vi "Rd Wr Focus settings json.vi"(7 "Focus Name":string="Default", 8 "error in (no error)":errorcluster, 9 "Settings File":string="CC System Settings.json", 10 "Write? (F:Read)":bool, 11 "Focus Settings":T1) -> (0 "error out":errorcluster, 3 "Focus Settings":T1)   [LabVIEW 2024]
uses:
  Focus cluster Settings.ctl
  Focus Hardware Types.ctl
  Focus cluster Motion Settings.ctl
  2e80df6d-94aa-46b9-8b94-ceea8c057880.vi
  659fb017-0e9f-42f9-b06e-930303f00cbc.vi
  <vilib>/JDP Science/JSONtext/Find Item.vi
  <vilib>/JDP Science/JSONtext/Next JSON Value.vi
  <vilib>/JDP Science/JSONtext/String Subset.vi
  <vilib>/JDP Science/JSONtext/Parsing/Advance past next JSON Value (inlined COPY).vi
  <vilib>/JDP Science/JSONtext/Parsing/Advance past whitespace.vi
  <vilib>/JDP Science/JSONtext/Parsing/Advance past String.vi
  <vilib>/JDP Science/JSONtext/Parsing/Advance past Number.vi
  <vilib>/JDP Science/JSONtext/Parsing/Advance past Line Ending.vi
  <vilib>/JDP Science/JSONtext/Parsing/Parse Full Path or Item Name.vi
  <vilib>/JDP Science/JSONtext/Parsing/Advance past Array.vi
  <vilib>/JDP Science/JSONtext/Parsing/Advance past Object.vi
  <vilib>/JDP Science/JSONtext/support/Error Cluster From Code.vi
  <vilib>/JDP Science/JSONtext/Offset/Find Item Locations by Path.vi
  <vilib>/JDP Science/JSONtext/JSON text to Variant.vi
  <vilib>/JDP Science/JSONtext/Variant to JSON Text.vi
  <vilib>/JDP Science/JSONtext/Set Item.vi
  <vilib>/JDP Science/JSONtext/LVClass Serializer/JSONtext LVClass Serializer.lvclass
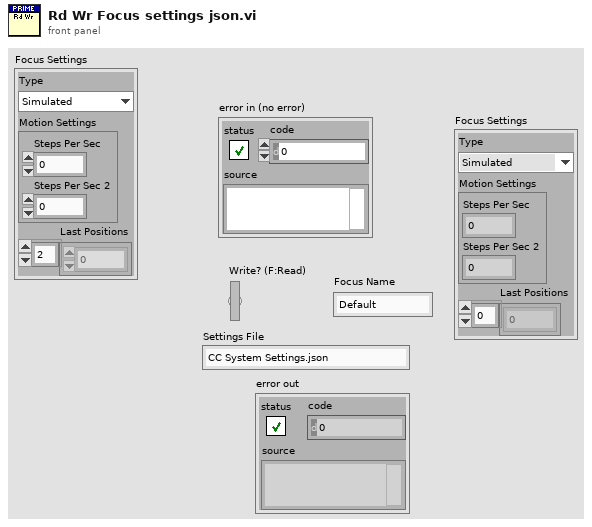
[diagram p1: front panel]
types:
  T1 = typedef "Focus cluster Settings.ctl" = cluster{"Type":T2, "Motion Settings":T3, "Last Positions":i32[]}
  T2 = typedef "Focus Hardware Types.ctl" = enum16{"Simulated", "NewFocus"}
  T3 = typedef "Focus cluster Motion Settings.ctl" = cluster{"Steps Per Sec":i32, "Steps Per Sec 2":i32}
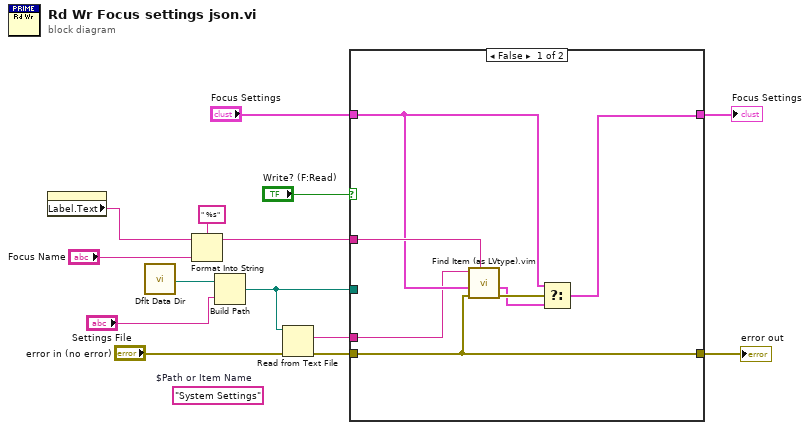
[diagram p0: block diagram]
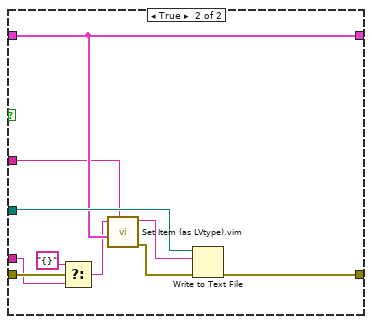
[diagram p2: hidden frame]
diagram:
  (unwired) "System Settings"  # $Path or Item Name
  n1 = property on="Focus Settings" class="Clust (strict)"() -> ("Label.Text"=w3:string)  [unwired: 2 in, 2 out]
  n2 = call <vilib>:"Dflt Data Dir.vi"() -> ("App:Default Data Directory"=w12:path)
  n3 = Format Into String(format string=" %s", initial string=w3, "Focus Name") -> (resulting string=w2:string)  [unwired: 1 in, 1 out]
  n4 = Build Path(base path=w12, name or relative path="Settings File") -> (appended path=w6:path)
  n5 = Read from Text File(file (use dialog)=w6, error in="error in (no error)") -> (text=w7:string, error out=w8:errorcluster)  [unwired: 2 in, 2 out]
  n6 = case shown="False" "Write? (F:Read)" {
    tunnel: w8 -> [w15 w26]
    tunnel: "Focus Settings" -> [w19 w29]
    tunnel: w6 -> [_ w31]
    tunnel: [w15 w30] -> w11
    tunnel: [w21 w29] -> w10
    tunnel: w2 -> [w20 w28]
    tunnel: w7 -> [w16 w24]
    frame False {
      n7 = call "Find Item (as LVtype).vim"("$Path or Item Name"=w20, "error in (no error)"=w15, "Data Type and Default Value"=w19, "JSON"=w16) -> ("error out"=w18:errorcluster, "Data"=w17:T1)  [unwired: 4 in, 2 out]
      n8 = Select(t=w19, s=w18, f=w17) -> (s? t:f=w21:T1)
    }
    frame True {
      n9 = Select(t="{}" ("JSON"), s=w26, f=w24) -> (s? t:f=w23:string)
      n10 = call "Set Item (as LVtype).vim"("$Path or Item Name"=w28, "Anything"=w29, "JSON"=w23) -> ("error out"=w22:errorcluster, "<JSON>"=w27:string)  [unwired: 5 in, 1 out]
      n11 = Write to Text File(file (use dialog)=w31, text=w27, error in=w22) -> (error out=w30:errorcluster)  [unwired: 1 in, 2 out]
    }
  }
  "error out" <- w11
  "Focus Settings" <- w10
